vi "RFmx MP Configuration.vi"(7 "Selector String":string, 8 "error in (no error)":errorcluster, 11 "Instrument Handle In":refnum<k21>) -> (0 "error out":errorcluster, 3 "Instrument Handle Out":refnum<k21>)   [LabVIEW 2018, in "DPD.lvlib"]
uses:
  DPD.lvlib
  Typedefs/Rfmx MP Configuration.ctl
panel:
  in  "RFmxMP Configuration":T1={"Mem Models Correction Type"=0, " Iterative DPD Enabled"=0, "Number of Iterations"=3, "Polynomial  Order"=3, "Memory Depth"=2, "Maximum Lag"=2, "Maximum Lead"=2, "Lag Order"=2, "Lead Order"=2, "Lag Memory Depth"=2, "Lead Memory Depth"=2} {"Number of Iterations" min=1; "Iterative DPD Enabled" items=["False", "True"]; "Mem Models Correction Type" items=["Magnitude and Phase", "Magnitude Only", "Phase Only"]}
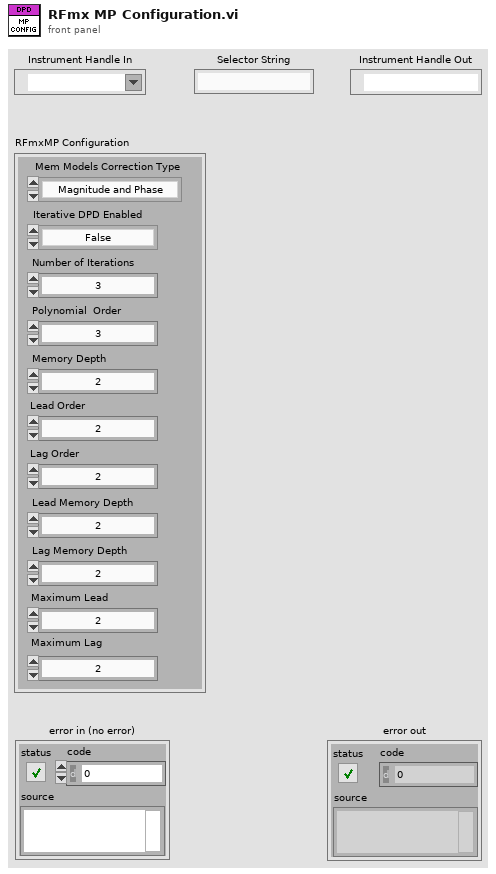
[diagram p1: front panel]
types:
  T1 = typedef "DPD.lvlib/Rfmx MP Configuration.ctl" = cluster{"Mem Models Correction Type":i32, " Iterative DPD Enabled":i32, "Number of Iterations":i32, "Polynomial  Order":i32, "Memory Depth":i32, "Maximum Lag":i32, "Maximum Lead":i32, "Lag Order":i32, "Lead Order":i32, "Lag Memory Depth":i32, "Lead Memory Depth":i32}
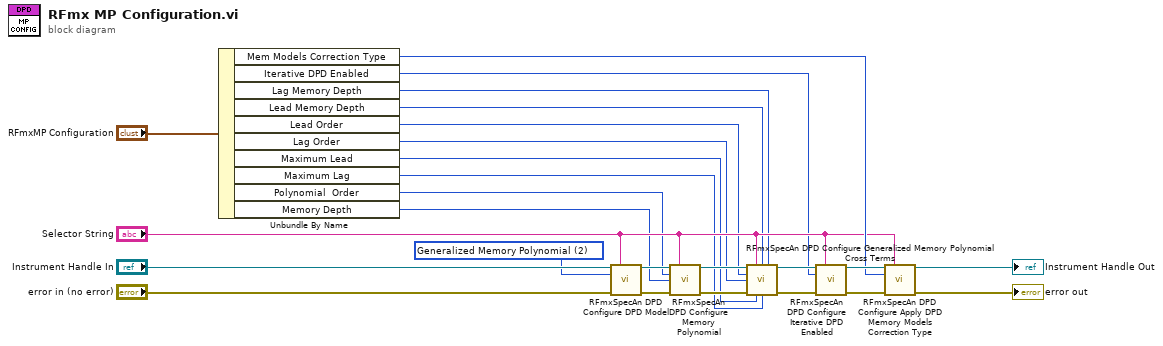
[diagram p0: block diagram]
diagram:
  w14 = 2 items=["Lookup Table", "Memory Polynomial", "Generalized Memory Polynomial"] ("DPD Model")
  n1 = Unbundle By Name("RFmxMP Configuration") -> ("Mem Models Correction Type"=w13:i32, "Iterative DPD Enabled"=w11:i32, "Lag Memory Depth"=w10:i32, "Lead Memory Depth"=w9:i32, "Lead Order"=w8:i32, "Lag Order"=w7:i32, "Maximum Lead"=w6:i32, "Maximum Lag"=w5:i32, "Polynomial  Order"=w4:i32, "Memory Depth"=w3:i32)
  n2 = call <vilib>:"RFmxSpecAn DPD Configure DPD Model.vi"("Instrument Handle In"="Instrument Handle In", "Selector String"="Selector String", "DPD Model"=w14, "error in (no error)"="error in (no error)") -> ("Instrument Handle Out"=w22:refnum<k21>, "error out"=w23:errorcluster)  [unwired: 10 in]
  n3 = call <vilib>:"RFmxSpecAn DPD Configure Memory Polynomial.vi"("Instrument Handle In"=w22, "Selector String"="Selector String", "Memory Polynomial Order"=w4, "Memory Polynomial Memory Depth"=w3, "error in (no error)"=w23) -> ("Instrument Handle Out"=w25:refnum<k21>, "error out"=w24:errorcluster)  [unwired: 9 in]
  n4 = call <vilib>:"RFmxSpecAn DPD Configure Generalized Memory Polynomial Cross Terms.vi"("Instrument Handle In"=w25, "Selector String"="Selector String", "Memory Polynomial Lead Memory Depth"=w9, "Memory Polynomial Lag Memory Depth"=w10, "Memory Polynomial Lead Order"=w8, "Memory Polynomial Lag Order"=w7, "error in (no error)"=w24, "Memory Polynomial Max Lead"=w6, "Memory Polynomial Max Lag"=w5) -> ("Instrument Handle Out"=w21:refnum<k21>, "error out"=w20:errorcluster)  [unwired: 5 in]
  n5 = call <vilib>:"RFmxSpecAn DPD Configure Iterative DPD Enabled.vi"("Instrument Handle In"=w21, "Selector String"="Selector String", "Iterative DPD Enabled"=w11, "error in (no error)"=w20) -> ("Instrument Handle Out"=w19:refnum<k21>, "error out"=w18:errorcluster)  [unwired: 10 in]
  n6 = call <vilib>:"RFmxSpecAn DPD Configure Apply DPD Memory Models Correction Type.vi"("Instrument Handle In"=w19, "Selector String"="Selector String", "Mem Models Correction Type"=w13, "error in (no error)"=w18) -> ("Instrument Handle Out"=→"Instrument Handle Out":refnum<k21>, "error out"=→"error out":errorcluster)  [unwired: 10 in]
